vi "Get Serial Port Timeout.vi"(8 "error in (no error)":errorcluster, 11 "VISA resource name":refnum<visa-resource-name>) -> (0 "error out":errorcluster, 2 "Timeout Value":dbl format="%.4f", 3 "VISA resource name out":refnum<visa-resource-name>)   [LabVIEW 2014, in "Fluke 5XXX Series Multicalibrators.lvlib"]
doc: "This VI returns the timeout period for the RS-232-C serial port. Timeout is the time the interface waits after being stalled before aborting the communication session.\n\nNote:\n\nThis VI is available only for instrument models 5700A and 5720A."
uses:
  Fluke 5XXX Series Multicalibrators.lvlib
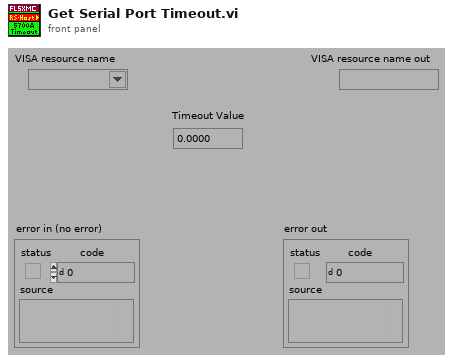
[diagram p1: front panel]
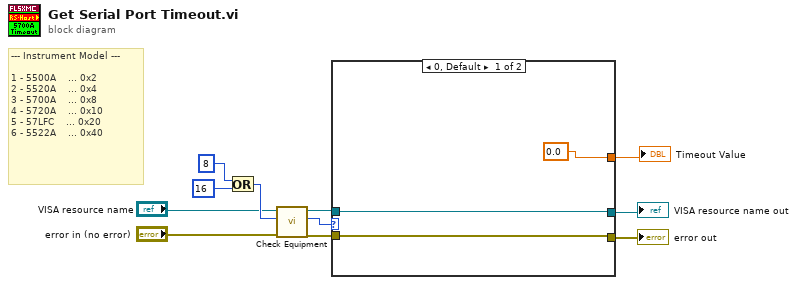
[diagram p0: block diagram]
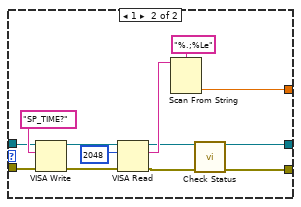
[diagram p2: hidden frame]
diagram:
  # "--- Instrument Model ---\n\n1 - 5500A    ... 0x2\n2 - 5520A    ... 0x4\n3 - 5700A    ... 0x8\n4 - 5720A    ... 0x10\n5 - 57LFC    ... 0x20\n6 - 5522A    ... 0x40"
  n1 = Or(x=8 ("Numeric"), y=16 ("Numeric")) -> (x .or. y?=w9:i32)
  n2 = call "Check Equipment.vi"("error in (no error)"="error in (no error)", "Bit Mask"=w9, "VISA resource name"="VISA resource name") -> ("error out"=w6:errorcluster, "Present?"=w4:u32, "VISA resource name out"=w5:refnum<visa-resource-name>)  [unwired: 6 in]
  n3 = case shown="0, Default" w4 {
    tunnel: [w14 w21] -> w3
    tunnel: [w13 w20] -> w2
    tunnel: w6 -> [w14 w23]
    tunnel: w5 -> [w13 w22]
    tunnel: [0.0 w17] -> w1
    frame 0, Default {
    }
    frame 1 {
      n4 = VISA Write(VISA resource name=w22, write buffer="SP_TIME?", error in (no error)=w23) -> (VISA resource name out=w26:refnum<visa-resource-name>, error out=w25:errorcluster)  [unwired: 1 out]
      n5 = VISA Read(VISA resource name=w26, byte count=u32 2048 ("byte count (0)"), error in (no error)=w25) -> (VISA resource name out=w15:refnum<visa-resource-name>, read buffer=w18:string, error out=w16:errorcluster)  [unwired: 1 out]
      n6 = Scan From String(format string="%.;%Le", input string=w18) -> (output 1=w17:dbl)  [unwired: 3 in, 3 out]
      n7 = call "Check Status.vi"("VISA resource name"=w15, "error in (no error)"=w16) -> ("VISA resource name out"=w20:refnum<visa-resource-name>, "error out"=w21:errorcluster)  [unwired: 12 in]
    }
  }
  "Timeout Value" <- w1
  "VISA resource name out" <- w2
  "error out" <- w3
